vi "read-islanding-ack.vi"() -> ()   [LabVIEW 2021]
panel:
  out "ack":T1
  in  "islanding-ack":string
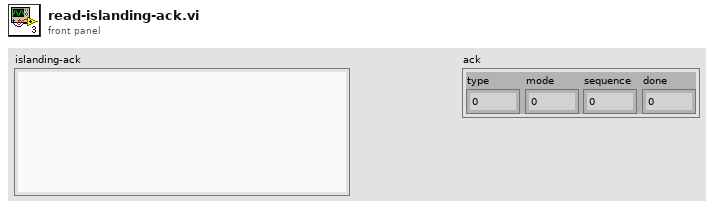
[diagram p1: front panel]
types:
  T1 = cluster{"type":dbl, "mode":dbl, "sequence":dbl, "done":dbl}
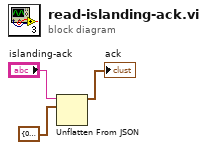
[diagram p0: block diagram]
diagram:
  n1 = Unflatten From JSON(JSON string="islanding-ack", type and defaults=T1 {"type"=0.0, "mode"=0.0, "sequence"=0.0, "done"=0.0} ("ack")) -> (value=→"ack":T1)  [unwired: 5 in, 1 out]
